vi "BatteryCyclingV1.0 Copy - Copy.vi"() -> ()   [LabVIEW 2020]
uses:
  <vilib>/addons/NHR/Public/Configure/Output Safety.ctl
  <vilib>/DAQmx/read.llb/DAQmx Read (Analog 1D DBL NChan 1Samp).vi
  <vilib>/DAQmx/miscellaneous.llb/DAQmx Fill In Error Info.vi
  <instrlib>/NH Research Regenerative Test Series/Public/Data/Read (Ave Current).vi
  <instrlib>/NH Research Regenerative Test Series/Public/Data/Low Level/Fetch (Ave Voltage).vi
  <instrlib>/NH Research Regenerative Test Series/Public/Data/Low Level/Fetch (Ave True Power).vi
  <instrlib>/NH Research Regenerative Test Series/NH Research Regenerative Test Series.lvlib
panel:
  out "Tab Control 2":T1(tab)
  out "Selected Output Safety 2":T2
  in  "Custom Output Safety 2":T2
  out "Discharge Rest Voltage":dbl(graph)
  out "Charge Rest Voltage":dbl(graph)
  out "Ave Current (A)":dbl
  out "Ave Voltage (V)":dbl
  out "Ave True Power (W)":dbl
  out "Battemp":dbl
  out "AmbientTemp":dbl
  in  "Tab Control":T1(tab)
  out "Selected Output Safety":T2
  in  "Custom Output Safety":T2
  in  "Output Safety\nSelection":bool caption="Output Safety"
  in  "Non Default Folder Path":path
  in  "Cycling Test Folder Name":string
  in  "DAQmx Task Name":refnum<k21>
  in  "NHR VISA Name":refnum<visa-resource-name>
  out "Error Out":string
  out "Previous Discharge Data File":path caption="Filename Out"
  out "Previous Charge Data File":path caption="Filename Out"
  out "D Wait Status Byte Register":T3
  out "Discharge Status Byte Register":T3
  out "C Wait Status Byte Register":T3
  out "Charge Status Byte Register":T3
  out "Task error out":errorcluster
  in  "Cycle Stop":bool
  out "Cycle Index":i32
  in  "Number of Cycles":i32
  out "Discharge Rest":bool
  in  "Wait Time":u32
  out "Discharge Rest Voltage":dbl
  out "Elaspsed Time":u32 caption="Elapsed Time (s)"
  out "Charge Rest":bool
  in  "Wait Time":u32
  out "Charge Rest Voltage":dbl
  out "Elapsed Time":u32 caption="Elapsed Time (s)"
  out "Discharging":bool
  in  "Discharge Stop":bool
  in  "Discharge Current":dbl
  in  "Voltage Cutoff":dbl
  out "Charging":bool
  in  "Charge Stop":bool
  in  "Current Cutoff":dbl
  in  "Charge Current":dbl format="%#.6g"
  in  "Charge Voltage":dbl format="%#.6g"
  in  "Logical Instrument Number":u32=1
  # "Rest Voltage Charts"
  # "Readings"
  # "Output Safety Configuration"
  # "Test Name & Device Info"
  # "Error Indication"
  # "Cycle & Charge Profile Settings"
  # "Cycle\nInfo"
  # "Post Discharge\nRest"
  # "Post Charge\nRest"
  # "Discharging"
  # "Charging"
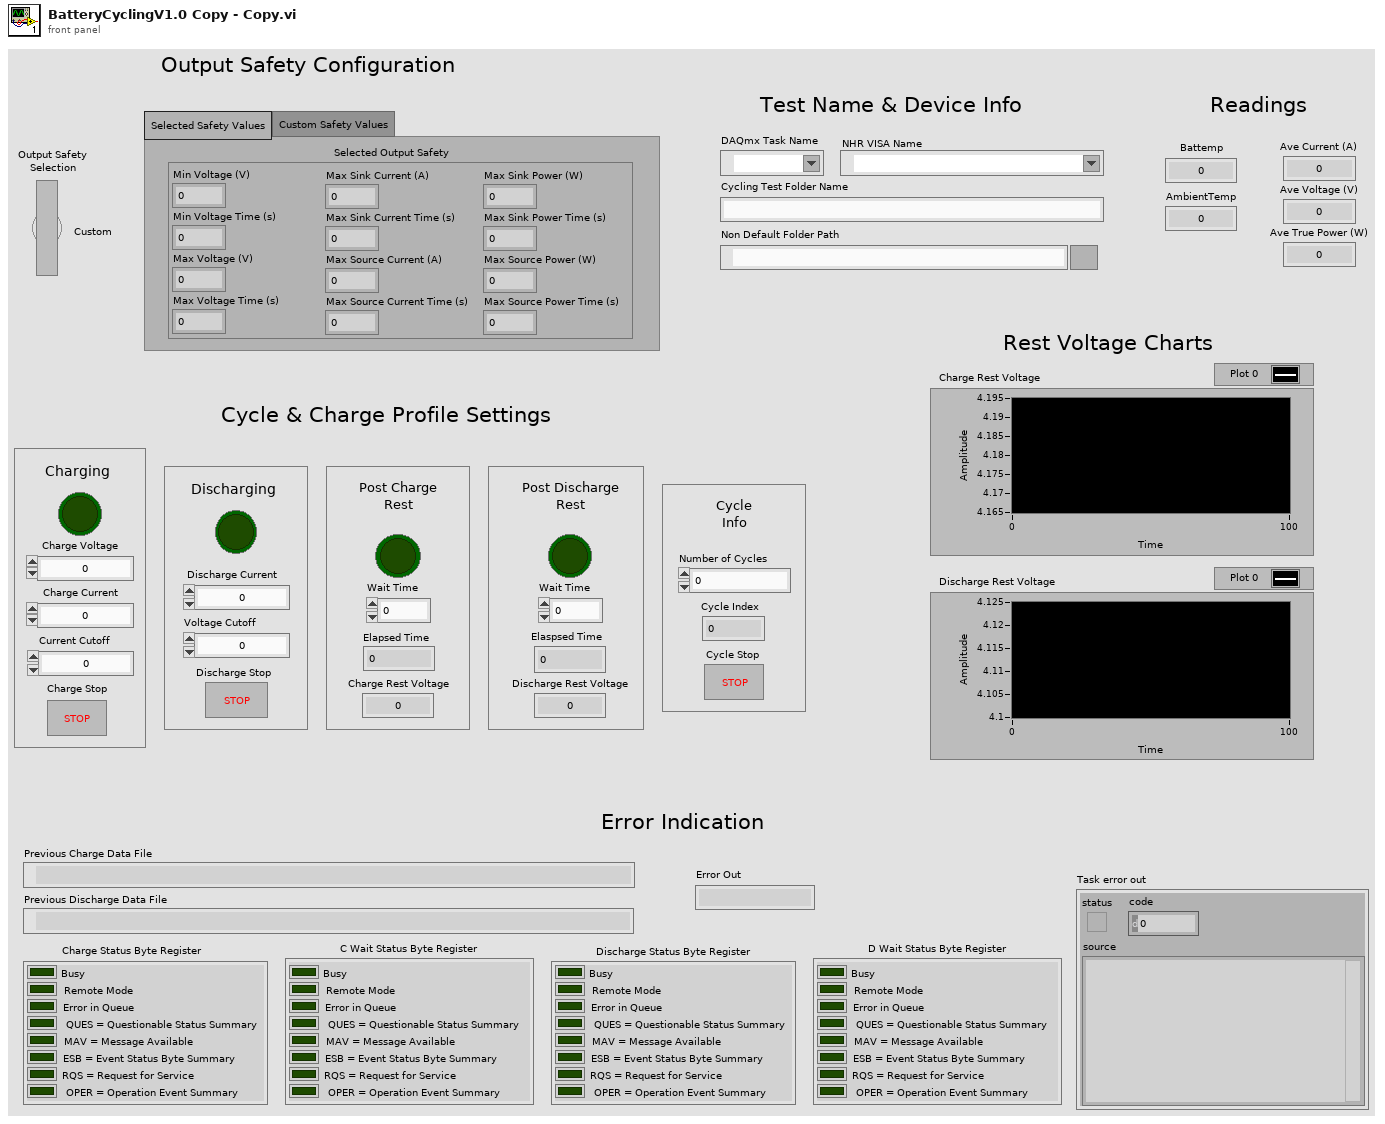
[diagram p1: front panel]
types:
  T1 = enum32{"Selected Safety Values", "Custom Safety Values"}
  T2 = typedef "NH Research Regenerative Test Series.lvlib/Output Safety.ctl" = cluster{"Min Voltage (V)":dbl, "Min Voltage Time (s)":dbl, "Max Voltage (V)":dbl, "Max Voltage Time (s)":dbl, "Max Sink Current (A)":dbl, "Max Sink Current Time (s)":dbl, "Max Source Current (A)":dbl, "Max Source Current Time (s)":dbl, "Max Sink Power (W)":dbl, "Max Sink Power Time (s)":dbl, "Max Source Power (W)":dbl, "Max Source Power Time (s)":dbl}
  T3 = cluster{"Busy":bool, "Remote Mode":bool, "Error in Queue":bool, "QUES = Questionable Status Summary":bool, "MAV = Message Available":bool, "ESB = Event Status Byte Summary":bool, "RQS = Request for Service":bool, "OPER = Operation Event Summary":bool}
  T4 = cluster{"Min Voltage (V)":dbl, "Min Voltage Time (s)":dbl, "Max Voltage (V)":dbl, "Max Voltage Time (s)":dbl, "Max Sink Current (A)":dbl, "Max Sink Current Time (s)":dbl, "Max Source Current (A)":dbl, "Max Source Current Time (s)":dbl, "Max Sink Power (W)":dbl, "Max Sink Power Time (s)":dbl, "Max Source Power (W)":dbl, "Max Source Power Time (s)":dbl}
  T5 = cluster{"data[0]":dbl, "data[1]":dbl, "data[2]":dbl, "data[3]":dbl, "data[4]":dbl, "data[5]":dbl, "data[6]":dbl, "data[7]":dbl, "data[8]":dbl}
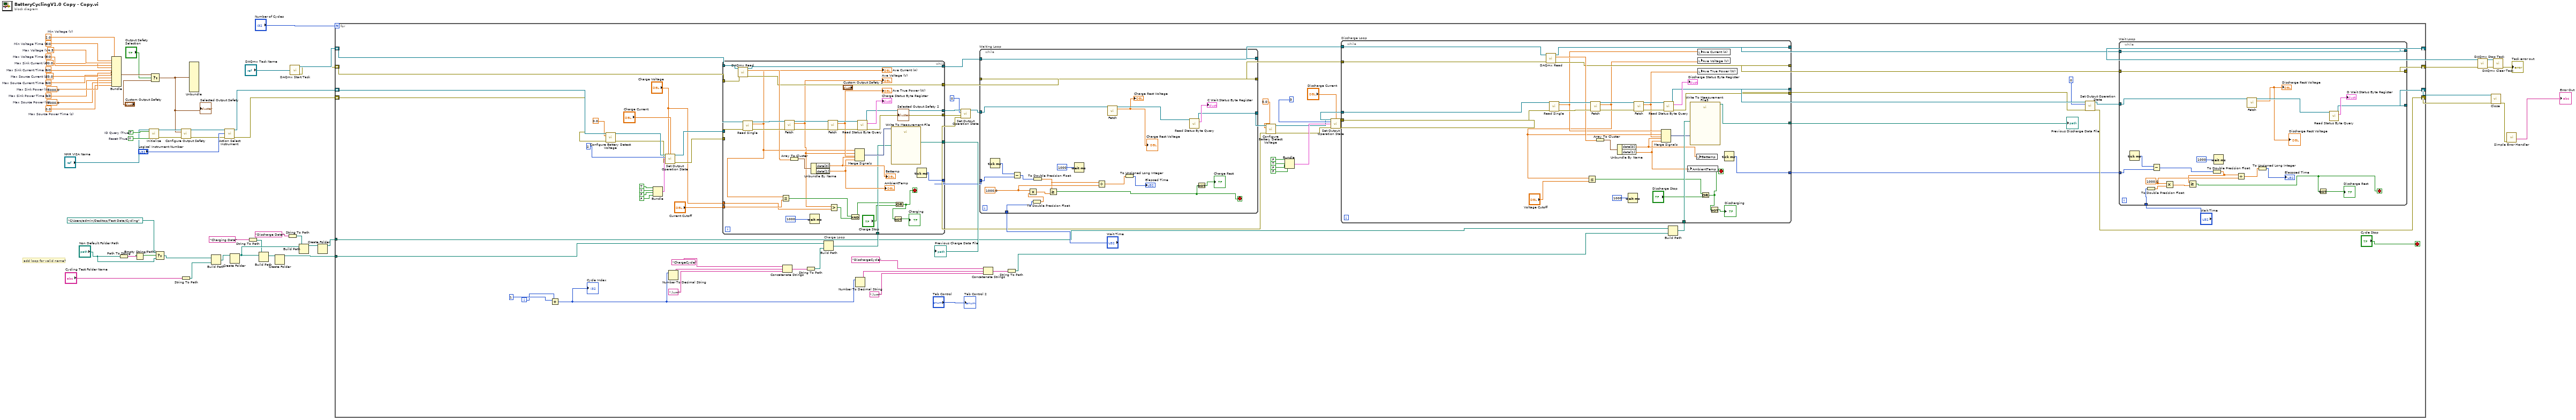
[diagram p0: block diagram]
diagram:
  w23 = 5000.0  # Max Source Power (W)
  w24 = 0.0  # Max Sink Power Time (s)
  w25 = 5000.0  # Max Sink Power (W)
  w26 = 0.0  # Max Source Current Time (s)
  w27 = 20.0  # Max Source Current (A)
  w29 = 20.0  # Max Sink Current (A)
  w28 = 0.0  # Max Sink Current Time (s)
  w30 = 0.0  # Max Voltage Time (s)
  w31 = 4.5  # Max Voltage (V)
  w32 = 2.0  # Min Voltage (V)
  w22 = 0.0  # Max Source Power Time (s)
  w33 = 0.0  # Min Voltage Time (s)
  w55 = TRUE  # ID Query (True)
  w54 = TRUE  # Reset (True)
  # "add loop for valid name?"
  n1 = Bundle("Min Voltage (V)"=w32, "Min Voltage Time (s)"=w33, "Max Voltage (V)"=w31, "Max Voltage Time (s)"=w30, "Max Sink Current (A)"=w29, "Max Sink Current Time (s)"=w28, "Max Source Current (A)"=w27, "Max Source Current Time (s)"=w26, "Max Sink Power (W)"=w25, "Max Sink Power Time (s)"=w24, "Max Source Power (W)"=w23, "Max Source Power Time (s)"=w22) -> (w20:T4)  [unwired: 1 in]
  n2 = Path To String(path="Non Default Folder Path") -> (string=w7:string)
  n3 = Empty String/Path?(string/path=w7) -> (empty?=w6:bool)
  n4 = call <instrlib>:"Initialize.vi"("VISA resource name"="NHR VISA Name", "ID Query (True)"=w55, "Reset (True)"=w54) -> ("VISA resource name out"=w53:refnum<visa-resource-name>, "error out"=w52:errorcluster)  [unwired: 11 in]
  n5 = Select(t=w20, s="Output Safety\nSelection", f="Custom Output Safety") -> (s? t:f=w21:T2)
  "Selected Output Safety" <- w21
  n6 = Select(t=path "C:/Users/admin/Desktop/Test Data/Cycling", s=w6, f="Non Default Folder Path") -> (s? t:f=w10:path)
  n7 = call <instrlib>:"Configure Output Safety.vi"("VISA resource name"=w53, "Output Safety"=w21, "error in (no error)"=w52) -> ("VISA resource name out"=w50:refnum<visa-resource-name>, "error out"=w46:errorcluster)  [unwired: 11 in]
  n8 = String To Path(string="Cycling Test Folder Name") -> (path=w12:path)
  n9 = Unbundle(w21) -> ()  [unwired: 12 out]
  n10 = Build Path(base path=w10, name or relative path=w12) -> (appended path=w9:path)
  n11 = call <instrlib>:"Action Select Instrument.vi"("VISA resource name"=w50, "Logical Instrument Number"="Logical Instrument Number", "error in (no error)"=w46) -> ("VISA resource name out"=w38:refnum<visa-resource-name>, "error out"=w37:errorcluster)  [unwired: 11 in]
  n12 = Create Folder(path (use dialog)=w9) -> (created path=w17:path)  [unwired: 2 in, 2 out]
  n13 = String To Path(string="Charging Data") -> (path=w13:path)
  n14 = Build Path(base path=w17, name or relative path=w13) -> (appended path=w14:path)
  n15 = Create Folder(path (use dialog)=w14) -> (created path=w1:path)  [unwired: 2 in, 2 out]
  n16 = String To Path(string="Discharge Data") -> (path=w15:path)
  n17 = call <vilib>:"DAQmx Start Task.vi"("task/channels in"="DAQmx Task Name") -> ("task out"=w48:refnum<k21>, "error out"=w47:errorcluster)  [unwired: 13 in]
  n18 = Build Path(base path=w17, name or relative path=w15) -> (appended path=w16:path)
  n19 = Create Folder(path (use dialog)=w16) -> (created path=w2:path)  [unwired: 2 in, 2 out]
  n20 = for {
    N: "Number of Cycles" -> [_]
    shift-right: [w82] -> w36
    shift-left: w38 -> [w93]
    shift-right: [w87] -> w35
    shift-left: w37 -> [w91]
    shift-right: [w80] -> w41
    shift-left: w48 -> [w130]
    shift-right: [w81] -> w40
    shift-left: w47 -> [w129]
    tunnel: w2 -> [w60]
    tunnel: w1 -> [w59]
    i -> [w88]
    stop <- "Cycle Stop" stop-if-true
    n21 = Add(x=1, y=w88) -> (x+y=w65:i32)
    "Cycle Index" <- w65
    n22 = call <instrlib>:"Configure Battery Detect Voltage.vi"("VISA resource name"=w93, "Battery Detect Voltage (0V)"=0.0, "error in (no error)"=w91) -> ("VISA resource name out"=w92:refnum<visa-resource-name>, "error out"=w90:errorcluster)  [unwired: 11 in]
    n23 = Bundle(TRUE, TRUE, FALSE, FALSE) -> (w94:cluster{bool, bool, bool, bool})  [unwired: 1 in]
    n24 = call <instrlib>:"Set Output Operation State.vi"("VISA resource name"=w92, "Voltage Setpoint (0 V)"="Charge Voltage", "Current Setpoint (0 A)"="Charge Current", "Mode (0: Off)"=2, "Enable"=w94, "error in (no error)"=w90) -> ("VISA resource name out"=w101:refnum<visa-resource-name>, "error out"=w100:errorcluster)  [unwired: 8 in]
    n25 = Number To Decimal String(number=w65) -> (decimal integer string=w74:string)  [unwired: 1 in]
    n26 = Concatenate Strings("ChargeCycle", w74, ".lvm") -> (w71:string)
    n27 = String To Path(string=w71) -> (path=w72:path)
    n28 = Build Path(base path=w59, name or relative path=w72) -> (appended path=w61:path)
    n29 = while "Charge Loop" {
      tunnel: w101 -> [w232]
      tunnel: w100 -> [w231]
      tunnel: [w229] -> w108
      tunnel: [w228] -> w107
      tunnel: "Current Cutoff" -> [w218]
      tunnel: w61 -> [w210]
      tunnel: w130 -> [w226]
      tunnel: [w222] -> w126
      tunnel: [w221] -> w125
      tunnel: w129 -> [w220]
      tunnel: [w219] -> w131
      tunnel: [w211] -> w78
      tunnel: "Charge Voltage" -> [w204]
      stop <- w207 stop-if-true
      n30 = call-poly <vilib>:"DAQmx Read.vi"("task/channels in"=w226, "error in"=w220) -> ("task out"=w222:refnum<k21>, "data"=w225:dbl[], "error out"=w221:errorcluster)  [unwired: 11 in]
      n31 = call-poly <instrlib>:"Read Single.vi"("VISA resource name"=w232, "error in (no error)"=w231) -> ("VISA resource name out"=w237:refnum<visa-resource-name>, "Ave Current (A)"=w215:dbl, "error out"=w238:errorcluster)  [unwired: 11 in]
      "Ave Current (A)" <- w215
      n32 = Less Or Equal?(x=w215, y=w218) -> (x <= y?=w213:bool)
      n33 = call-poly <instrlib>:"Fetch.vi"("VISA resource name"=w237, "error in (no error)"=w238) -> ("VISA resource name out"=w236:refnum<visa-resource-name>, "Ave Voltage (V)"=w205:dbl, "error out"=w235:errorcluster)  [unwired: 11 in]
      "Ave Voltage (V)" <- w205
      n34 = Array To Cluster(array=w225) -> (cluster=w224:T5)
      n35 = Wait (ms)(milliseconds to wait=1000) -> ()  [unwired: 1 out]
      n36 = Unbundle By Name(w224) -> ("data[0]"=w217:dbl, "data[1]"=w216:dbl)
      "Battemp" <- w217
      "AmbientTemp" <- w216
      n37 = call-poly <instrlib>:"Fetch.vi"("VISA resource name"=w236, "error in (no error)"=w235) -> ("VISA resource name out"=w234:refnum<visa-resource-name>, "Ave True Power (W)"=w227:dbl, "error out"=w233:errorcluster)  [unwired: 11 in]
      "Ave True Power (W)" <- w227
      n38 = Greater?(x=w205, y=w204) -> (0:w212:bool)
      n39 = And(x=w213, y=w212) -> (x .and. y?=w209:bool)
      n40 = Merge Signals "Merge Signals"(w215, w205, w227, w217, w216) -> (w223:dynamicdata)
      n41 = call <instrlib>:"Read Status Byte Query.vi"("VISA resource name"=w234, "error in (no error)"=w233) -> ("VISA resource name out"=w229:refnum<visa-resource-name>, "Status Byte Register"=→"Charge Status Byte Register":T3, "error out"=w228:errorcluster)  [unwired: 11 in]
      n42 = call "Write To Measurement File"("Signals"=w223, "Filename"=w210) -> ("Filename Out"=w219:path)  [unwired: 15 in, 2 out]
      n43 = Or(x=w209, y="Charge Stop") -> (x .or. y?=w207:bool)
      n44 = Not(x=w207) -> (.not. x?=→"Charging":bool)
      n45 = Tick Count (ms)() -> (millisecond timer value=w211:u32)
    }
    "Previous Charge Data File" <- w131
    n46 = Number To Decimal String(number=w65) -> (decimal integer string=w69:string)  [unwired: 1 in]
    n47 = call <instrlib>:"Set Output Operation State.vi"("VISA resource name"=w108, "Mode (0: Off)"=0, "error in (no error)"=w107) -> ("VISA resource name out"=w104:refnum<visa-resource-name>, "error out"=w106:errorcluster)  [unwired: 11 in]
    n48 = while "Waiting Loop" {
      tunnel: [w202] -> w110
      tunnel: "Wait Time" -> [w185]
      tunnel: w78 -> [w199]
      tunnel: [w195] -> w121
      tunnel: [w196] -> w122
      tunnel: w125 -> [w195]
      tunnel: w126 -> [w196]
      tunnel: w104 -> [w194]
      stop <- w191 stop-if-true
      w200 = 1000.0
      n49 = Tick Count (ms)() -> (millisecond timer value=w198:u32)
      n50 = Subtract(x=w198, y=w199) -> (x-y=w187:u32)
      n51 = To Double Precision Float(number=w185) -> (double precision float=w184:dbl)
      n52 = Multiply(x=w200, y=w184) -> (x*y=w201:dbl)
      n53 = To Double Precision Float(number=w187) -> (double precision float=w186:dbl)
      n54 = Greater Or Equal?(x=w186, y=w201) -> (x >= y?=w191:bool)
      n55 = Wait (ms)(milliseconds to wait=1000) -> ()  [unwired: 1 out]
      n56 = Divide(x=w186, y=w200) -> (x/y=w189:dbl)
      n57 = call-poly <instrlib>:"Fetch.vi"("VISA resource name"=w194) -> ("VISA resource name out"=w193:refnum<visa-resource-name>, "Ave Voltage (V)"=→"Charge Rest Voltage" →"Charge Rest Voltage":dbl)  [unwired: 12 in, 1 out]
      n58 = To Unsigned Long Integer(number=w189) -> (unsigned 32bit integer=→"Elapsed Time":u32)
      n59 = call <instrlib>:"Read Status Byte Query.vi"("VISA resource name"=w193) -> ("VISA resource name out"=w202:refnum<visa-resource-name>, "Status Byte Register"=→"C Wait Status Byte Register":T3)  [unwired: 12 in, 1 out]
      n60 = Not(x=w191) -> (.not. x?=→"Charge Rest":bool)
    }
    n61 = Concatenate Strings("DischargeCycle", w69, ".lvm") -> (w67:string)
    n62 = String To Path(string=w67) -> (path=w64:path)
    n63 = call <instrlib>:"Configure Battery Detect Voltage.vi"("VISA resource name"=w110, "Battery Detect Voltage (0V)"=0.0, "error in (no error)"=w106) -> ("VISA resource name out"=w109:refnum<visa-resource-name>, "error out"=w111:errorcluster)  [unwired: 11 in]
    n64 = Bundle(FALSE, TRUE, FALSE, FALSE) -> (w116:cluster{bool, bool, bool, bool})  [unwired: 1 in]
    n65 = call <instrlib>:"Set Output Operation State.vi"("VISA resource name"=w109, "Current Setpoint (0 A)"="Discharge Current", "Mode (0: Off)"=3, "Enable"=w116, "error in (no error)"=w111) -> ("VISA resource name out"=w123:refnum<visa-resource-name>, "error out"=w124:errorcluster)  [unwired: 9 in]
    n66 = Build Path(base path=w60, name or relative path=w64) -> (appended path=w76:path)
    n67 = while "Discharge Loop" {
      tunnel: w123 -> [w177]
      tunnel: w124 -> [w176]
      tunnel: [w174] -> w114
      tunnel: [w173] -> w113
      tunnel: w76 -> [w172]
      tunnel: w122 -> [w171]
      tunnel: [w167] -> w85
      tunnel: [w166] -> w84
      tunnel: w121 -> [w165]
      tunnel: [w164] -> w86
      tunnel: [w162] -> w77
      stop <- w157 stop-if-true
      n68 = call-poly <vilib>:"DAQmx Read.vi"("task/channels in"=w171, "error in"=w165) -> ("task out"=w167:refnum<k21>, "data"=w170:dbl[], "error out"=w166:errorcluster)  [unwired: 11 in]
      n69 = call-poly <instrlib>:"Read Single.vi"("VISA resource name"=w177, "error in (no error)"=w176) -> ("VISA resource name out"=w182:refnum<visa-resource-name>, "Ave Current (A)"=w154:dbl, "error out"=w183:errorcluster)  [unwired: 11 in]
      n70 = call-poly <instrlib>:"Fetch.vi"("VISA resource name"=w182, "error in (no error)"=w183) -> ("VISA resource name out"=w181:refnum<visa-resource-name>, "Ave Voltage (V)"=w153:dbl, "error out"=w180:errorcluster)  [unwired: 11 in]
      n71 = Less Or Equal?(x=w153, y="Voltage Cutoff") -> (x <= y?=w160:bool)
      n72 = Array To Cluster(array=w170) -> (cluster=w169:T5)
      n73 = Unbundle By Name(w169) -> ("data[0]"=w156:dbl, "data[1]"=w155:dbl)
      n74 = Wait (ms)(milliseconds to wait=1000) -> ()  [unwired: 1 out]
      n75 = call-poly <instrlib>:"Fetch.vi"("VISA resource name"=w181, "error in (no error)"=w180) -> ("VISA resource name out"=w179:refnum<visa-resource-name>, "Ave True Power (W)"=w152:dbl, "error out"=w178:errorcluster)  [unwired: 11 in]
      n76 = Merge Signals "Merge Signals"(w154, w153, w152, w156, w155) -> (w168:dynamicdata)
      n77 = call <instrlib>:"Read Status Byte Query.vi"("VISA resource name"=w179, "error in (no error)"=w178) -> ("VISA resource name out"=w174:refnum<visa-resource-name>, "Status Byte Register"=→"Discharge Status Byte Register":T3, "error out"=w173:errorcluster)  [unwired: 11 in]
      n78 = local write "AmbientTemp"(w155) -> ()
      n79 = call "Write To Measurement File3"("Signals"=w168, "Filename"=w172) -> ("Filename Out"=w164:path)  [unwired: 15 in, 2 out]
      n80 = local write "Battemp"(w156) -> ()
      n81 = local write "Ave Current (A)"(w154) -> ()
      n82 = local write "Ave Voltage (V)"(w153) -> ()
      n83 = local write "Ave True Power (W)"(w152) -> ()
      n84 = Or(x=w160, y="Discharge Stop") -> (x .or. y?=w157:bool)
      n85 = Not(x=w157) -> (.not. x?=→"Discharging":bool)
      n86 = Tick Count (ms)() -> (millisecond timer value=w162:u32)
    }
    "Previous Discharge Data File" <- w86
    n87 = call <instrlib>:"Set Output Operation State.vi"("VISA resource name"=w114, "Mode (0: Off)"=0, "error in (no error)"=w113) -> ("VISA resource name out"=w83:refnum<visa-resource-name>, "error out"=w87:errorcluster)  [unwired: 11 in]
    n88 = while "Wait Loop" {
      tunnel: [w150] -> w82
      tunnel: "Wait Time" -> [w134]
      tunnel: w77 -> [w147]
      tunnel: [w144] -> w81
      tunnel: [w145] -> w80
      tunnel: w84 -> [w144]
      tunnel: w85 -> [w145]
      tunnel: w83 -> [w143]
      stop <- w138 stop-if-true
      w148 = 1000.0
      n89 = Tick Count (ms)() -> (millisecond timer value=w146:u32)
      n90 = To Double Precision Float(number=w134) -> (double precision float=w133:dbl)
      n91 = Subtract(x=w146, y=w147) -> (x-y=w141:u32)
      n92 = Multiply(x=w148, y=w133) -> (x*y=w149:dbl)
      n93 = To Double Precision Float(number=w141) -> (double precision float=w132:dbl)
      n94 = Greater Or Equal?(x=w132, y=w149) -> (x >= y?=w138:bool)
      n95 = Wait (ms)(milliseconds to wait=u32 1000) -> ()  [unwired: 1 out]
      n96 = Divide(x=w132, y=w148) -> (x/y=w136:dbl)
      n97 = call-poly <instrlib>:"Fetch.vi"("VISA resource name"=w143) -> ("VISA resource name out"=w142:refnum<visa-resource-name>, "Ave Voltage (V)"=→"Discharge Rest Voltage" →"Discharge Rest Voltage":dbl)  [unwired: 12 in, 1 out]
      n98 = To Unsigned Long Integer(number=w136) -> (unsigned 32bit integer=→"Elaspsed Time":u32)
      n99 = Not(x=w138) -> (.not. x?=→"Discharge Rest":bool)
      n100 = call <instrlib>:"Read Status Byte Query.vi"("VISA resource name"=w142) -> ("VISA resource name out"=w150:refnum<visa-resource-name>, "Status Byte Register"=→"D Wait Status Byte Register":T3)  [unwired: 12 in, 1 out]
    }
    "Tab Control 2" <- "Tab Control"
  }
  n101 = call <vilib>:"DAQmx Stop Task.vi"("task/channels in"=w41, "error in"=w40) -> ("task out"=w45:refnum<k21>, "error out"=w44:errorcluster)  [unwired: 12 in]
  n102 = call <instrlib>:"Close.vi"("VISA resource name"=w36, "error in (no error)"=w35) -> ("error out"=w42:errorcluster)  [unwired: 13 in]
  n103 = call <vilib>:"DAQmx Clear Task.vi"("task in"=w45, "error in"=w44) -> ("error out"=→"Task error out":errorcluster)  [unwired: 13 in]
  n104 = call <vilib>:"Simple Error Handler.vi"("error in (no error)"=w42) -> ("source out"=→"Error Out":string)  [unwired: 4 in, 4 out]
